vi "hw2p6_hickey.vi"() -> ()   [LabVIEW 2014]
panel:
  in  "stop":bool
  out "Odd":bool
  out "Even":bool
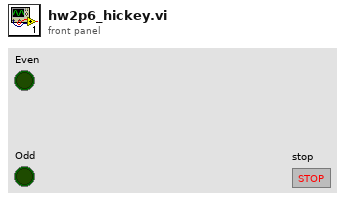
[diagram p1: front panel]
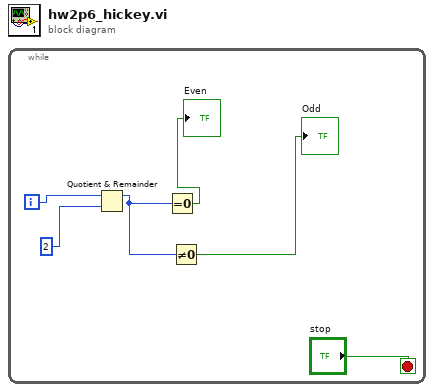
[diagram p0: block diagram]
diagram:
  n1 = while {
    i -> [w5]
    stop <- "stop" stop-if-true
    n2 = Quotient & Remainder(x=w5, y=2) -> (x-y*floor(x/y)=w2:i32)  [unwired: 1 out]
    n3 = Equal To 0?(x=w2) -> (x = 0?=→"Even":bool)
    n4 = Not Equal To 0?(x=w2) -> (x != 0?=→"Odd":bool)
  }
